vi "ElapsedTime.vi"(8 "error in (no error)":errorcluster, 10 "Mode (Update)":enum16{"Update", "Init"}(ring)) -> (0 "error out":errorcluster, 2 "Elapsed Time":dbl)   [LabVIEW 2013]
doc: "Use this template to build a VI to use as a subVI."
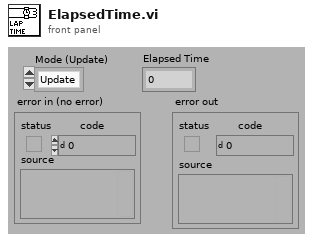
[diagram p1: front panel]
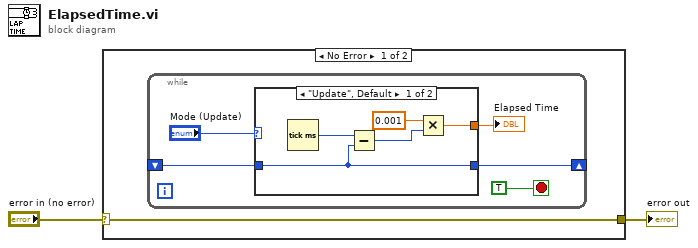
[diagram p0: block diagram]
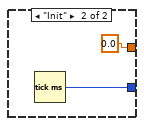
[diagram p2: hidden frame]
diagram:
  n1 = case shown="No Error" "error in (no error)" {
    selector: "error in (no error)" -> [w3 w16]
    tunnel: [w3 w16] -> w1
    frame No Error {
      n2 = while {
        shift-right: [w7] -> _
        shift-left: _ -> [w6]
        stop <- TRUE stop-if-true
        n3 = case shown="\"Update\", Default" "Mode (Update)" {
          tunnel: w6 -> [w12 _]
          tunnel: [w12 w15] -> w7
          tunnel: [w11 0.0] -> w5
          frame "Update", Default {
            n4 = Tick Count (ms)() -> (millisecond timer value=w13:u32)
            n5 = Subtract(x=w13, y=w12) -> (x-y=w9:u32)
            n6 = Multiply(x=0.001, y=w9) -> (x*y=w11:dbl)
          }
          frame "Init" {
            n7 = Tick Count (ms)() -> (millisecond timer value=w15:u32)
          }
        }
        "Elapsed Time" <- w5
      }
    }
    frame Error {
    }
  }
  "error out" <- w1
